vi "Get Value List.vi"(8 "error in (no error)":errorcluster, 10 "Indice de fila":i32, 11 "Soda Actor in":refnum<class "Soda Actor.lvclass">) -> (0 "error out":errorcluster, 3 "Soda Actor out":refnum<class "Soda Actor.lvclass">)   [LabVIEW 2020, in "Soda Actor.lvlib" / "Soda Actor.lvclass"]
uses:
  Soda Actor.lvclass
  C:/Program Files (x86)/National Instruments/LabVIEW 2020/vi.lib/ActorFramework/Actor/Actor.lvclass
  <vilib>/ActorFramework/Actor/Actor.lvclass/Actor.ctl
  Soda Actor.lvclass/Soda Actor.ctl
  UI Actor Messages/Update Values Msg/Update Values Msg.lvclass/Update Values Msg.ctl
  <vilib>/ActorFramework/Message Enqueuer/Message Enqueuer.lvclass/Message Enqueuer.ctl
  <vilib>/ActorFramework/Message Enqueuer/Enqueue.vi
  UI Actor Messages/Update Values Msg/Update Values Msg.lvclass
  C:/Program Files (x86)/National Instruments/LabVIEW 2020/vi.lib/ActorFramework/Message/Message.lvclass
  <vilib>/ActorFramework/Message Priority Queue/Priority Enqueue.vi
  <vilib>/ActorFramework/Actor/Actor.lvclass
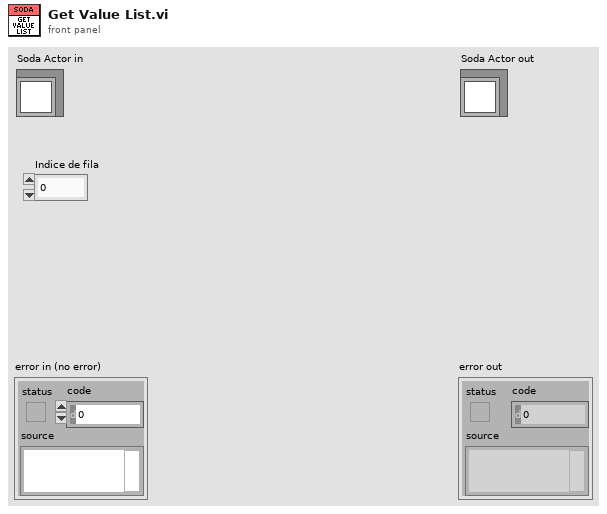
[diagram p1: front panel]
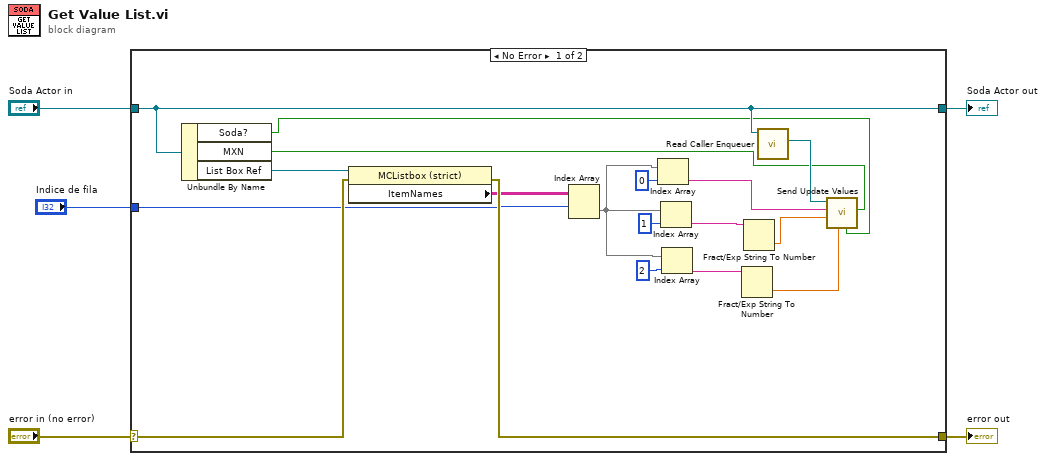
[diagram p0: block diagram]
diagram:
  n1 = case shown="No Error" "error in (no error)" {
    selector: "error in (no error)" -> [w22 w25]
    tunnel: [w21 w25] -> w4
    tunnel: [w14 w24] -> w2
    tunnel: "Soda Actor in" -> [w14 w24]
    tunnel: "Indice de fila" -> [w19 _]
    frame No Error {
      n2 = Unbundle By Name(w14) -> ("Soda?"=w6:bool, "MXN"=w7:bool, "List Box Ref"=w23:refnum<vi>)
      n3 = property class="MCListbox (strict)"(reference=w23, error in=w22) -> (error out=w21:errorcluster, "ItemNames"=w20:string[][])  [unwired: 1 out]
      n4 = Index Array(array=w20, index (row)=w19) -> (element=w15:string[])  [unwired: 1 in]
      n5 = Index Array(array=w15, index=0 ("index (row)")) -> (element=w12:string)
      n6 = Index Array(array=w15, index=1 ("index (row)")) -> (element=w9:string)
      n7 = Index Array(array=w15, index=2 ("index (row)")) -> (element=w11:string)
      n8 = Fract/Exp String To Number(string=w11) -> (number=w10:dbl)  [unwired: 3 in, 1 out]
      n9 = Fract/Exp String To Number(string=w9) -> (number=w8:dbl)  [unwired: 3 in, 1 out]
      n10 = call <vilib>:"Read Caller Enqueuer.vi"("Actor"=w14) -> ("Caller Enqueuer"=w13:refnum<class "Message Enqueuer.lvclass">)  [unwired: 10 in]
      n11 = call "Send Update Values.vi"("MXN?"=w7, "Soda?"=w6, "Inventario"=w10, "Costo"=w8, "Producto"=w12, "Message Enqueuer"=w13) -> ()  [unwired: 4 in, 2 out]
    }
    frame Error {
    }
  }
  "error out" <- w4
  "Soda Actor out" <- w2
